vi "GetQueuePosConfigFromQueue.vi"(8 "error in (no error)":errorcluster, 11 "ParameterConf in":refnum<class "ParameterConf.lvclass">) -> (0 "error out":errorcluster, 2 "element":T2, 3 "ParameterConf out":refnum<class "ParameterConf.lvclass">)   [LabVIEW 2014, in "LibraryGcode.lvlib" / "ParameterConf.lvclass"]
uses:
  ParameterConf.lvclass
  control/stateCmdUpdatePara.ctl
  ParameterConf.lvclass/ParameterConf.ctl
  LibraryGcode.lvlib
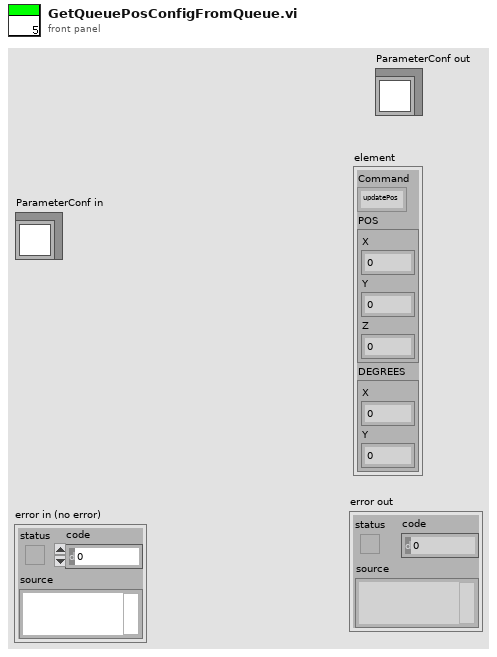
[diagram p1: front panel]
types:
  T1 = typedef "LibraryGcode.lvlib/stateCmdUpdatePara.ctl" = enum16{"updatePos", "UpdateConfigAccel", "UpdateConfigFeed", "UpdateConfigUnit", "UpdateConfigStartAccel", "NoUpdate"}
  T2 = cluster{"Command":T1, "POS":cluster{"X":dbl, "Y":dbl, "Z":dbl}, "DEGREES":cluster{"X":dbl, "Y":dbl}}
  T3 = typedef "LibraryGcode.lvlib/TypeDataPOS.ctl" = cluster{"Command":T1, "POS":cluster{"X":dbl, "Y":dbl, "Z":dbl}, "DEGREES":cluster{"X":dbl, "Y":dbl}}
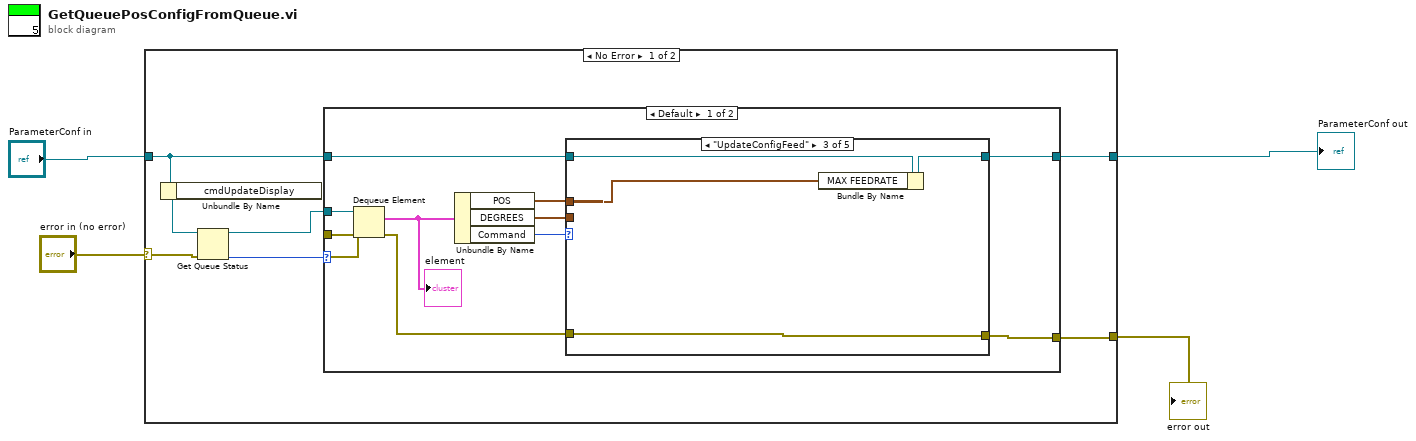
[diagram p0: block diagram]
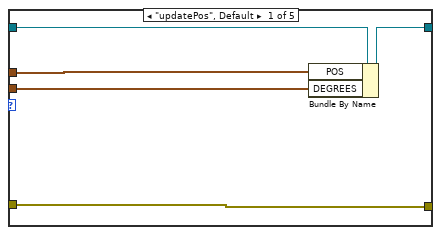
[diagram p2: hidden frame]
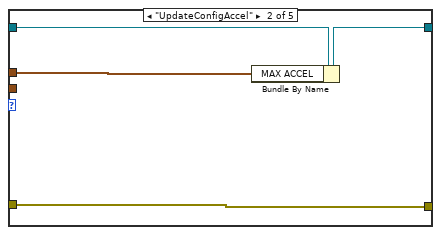
[diagram p3: hidden frame]
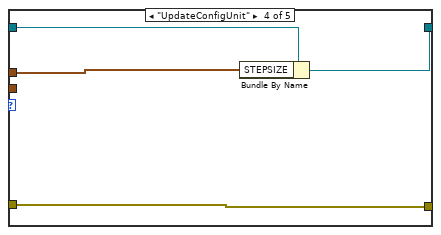
[diagram p4: hidden frame]
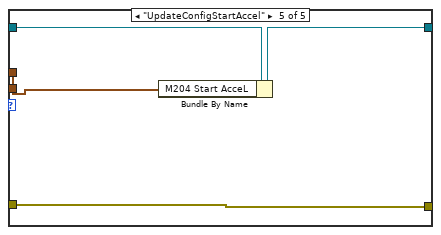
[diagram p5: hidden frame]
diagram:
  n1 = case shown="No Error" "error in (no error)" {
    selector: "error in (no error)" -> [w10 w47]
    tunnel: [w6 w47] -> w2
    tunnel: [w7 w46] -> w1
    tunnel: "ParameterConf in" -> [w8 w46]
    frame No Error {
      n2 = Unbundle By Name(w8) -> ("cmdUpdateDisplay"=w11:refnum<queue>)
      n3 = Get Queue Status(queue=w11, error in (no error)=w10) -> (queue out=w5:refnum<queue>, error out=w9:errorcluster, # elements in queue=w12:i32)  [unwired: 1 in, 5 out]
      n4 = case shown="Default" w12 {
        tunnel: w5 -> [w16 _]
        tunnel: w9 -> [w22 w44]
        tunnel: w8 -> [w20 w45]
        tunnel: [w19 w45] -> w7
        tunnel: [w17 w44] -> w6
        frame Default {
          n5 = Dequeue Element(queue=w16, error in (no error)=w22) -> (element=w15:T3, error out=w18:errorcluster)  [unwired: 1 in, 2 out]
          "element" <- w15
          n6 = Unbundle By Name(w15) -> ("POS"=w21:cluster{"X":dbl, "Y":dbl, "Z":dbl}, "DEGREES"=w14:cluster{"X":dbl, "Y":dbl}, "Command"=w13:T1)
          n7 = case shown="\"UpdateConfigFeed\"" w13 {
            tunnel: w21 -> [w27 w29 w33 w38 w43]
            tunnel: w14 -> [w26 _ _ _ _]
            tunnel: [w24 w30 w34 w39 w42] -> w19
            tunnel: w20 -> [w25 w31 w35 w37 w41]
            tunnel: [w23 w28 w32 w36 w40] -> w17
            tunnel: w18 -> [w23 w28 w32 w36 w40]
            frame "updatePos", Default {
              n8 = Bundle By Name(cluster=w25, "POS"=w27, "DEGREES"=w26) -> (w24:refnum<class "ParameterConf.lvclass">)
            }
            frame "UpdateConfigAccel" {
              n9 = Bundle By Name(cluster=w31, "MAX ACCEL"=w29) -> (w30:refnum<class "ParameterConf.lvclass">)
            }
            frame "UpdateConfigFeed" {
              n10 = Bundle By Name(cluster=w35, "MAX FEEDRATE"=w33) -> (w34:refnum<class "ParameterConf.lvclass">)
            }
            frame "UpdateConfigUnit" {
              n11 = Bundle By Name(cluster=w37, "STEPSIZE"=w38) -> (w39:refnum<class "ParameterConf.lvclass">)
            }
            frame "UpdateConfigStartAccel" {
              n12 = Bundle By Name(cluster=w41, "M204 Start AcceL"=w43) -> (w42:refnum<class "ParameterConf.lvclass">)
            }
          }
        }
        frame 0 {
        }
      }
    }
    frame Error {
    }
  }
  "ParameterConf out" <- w1
  "error out" <- w2
